vi "Current autoranger.vi"(1 "Current (µA)":dbl) -> (0 "Range":string)   [LabVIEW 2015]
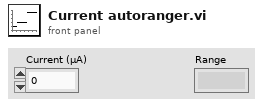
[diagram p1: front panel]
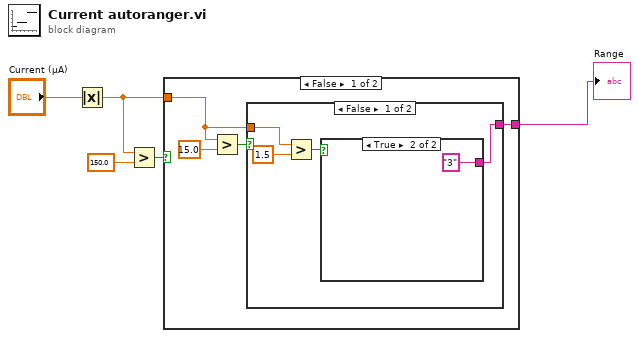
[diagram p0: block diagram]
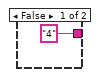
[diagram p2: hidden frame]
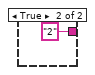
[diagram p3: hidden frame]
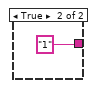
[diagram p4: hidden frame]
diagram:
  n1 = Absolute Value(x="Current (µA)") -> (abs(x)=w3:dbl)
  n2 = Greater?(x=w3, y=150.0) -> (0:w5:bool)
  n3 = case shown="False" w5 {
    tunnel: w3 -> [w7 _]
    tunnel: [w6 "1"] -> w1
    frame False {
      n4 = Greater?(x=w7, y=15.0) -> (0:w8:bool)
      n5 = case shown="False" w8 {
        tunnel: w7 -> [w12 _]
        tunnel: [w10 "2"] -> w6
        frame False {
          n6 = Greater?(x=w12, y=1.5) -> (0:w11:bool)
          n7 = case shown="True" w11 {
            tunnel: ["4" "3"] -> w10
            frame False {
            }
            frame True {
            }
          }
        }
        frame True {
        }
      }
    }
    frame True {
    }
  }
  "Range" <- w1
